vi "Start.vi"(8 "error in (no error)":errorcluster, 9 "Channel Data (DBLs Only)":T1, 10 "Real-Time System Data":T2, 11 "Configuration Data":T3) -> (0 "error out":errorcluster, 1 "Channel Data (DBLs Only)":T1, 2 "Real-Time System Data":T2, 3 "Configuration Data":T3)   [LabVIEW 2014, in "RM interrupt timing Custom Device.lvlib"]
uses:
  RM interrupt timing Custom Device.lvlib
  Configuration Data.ctl
  Real-Time System Data.ctl
  Channel Data.ctl
panel:
  # "Controls"
  # "Indicators"
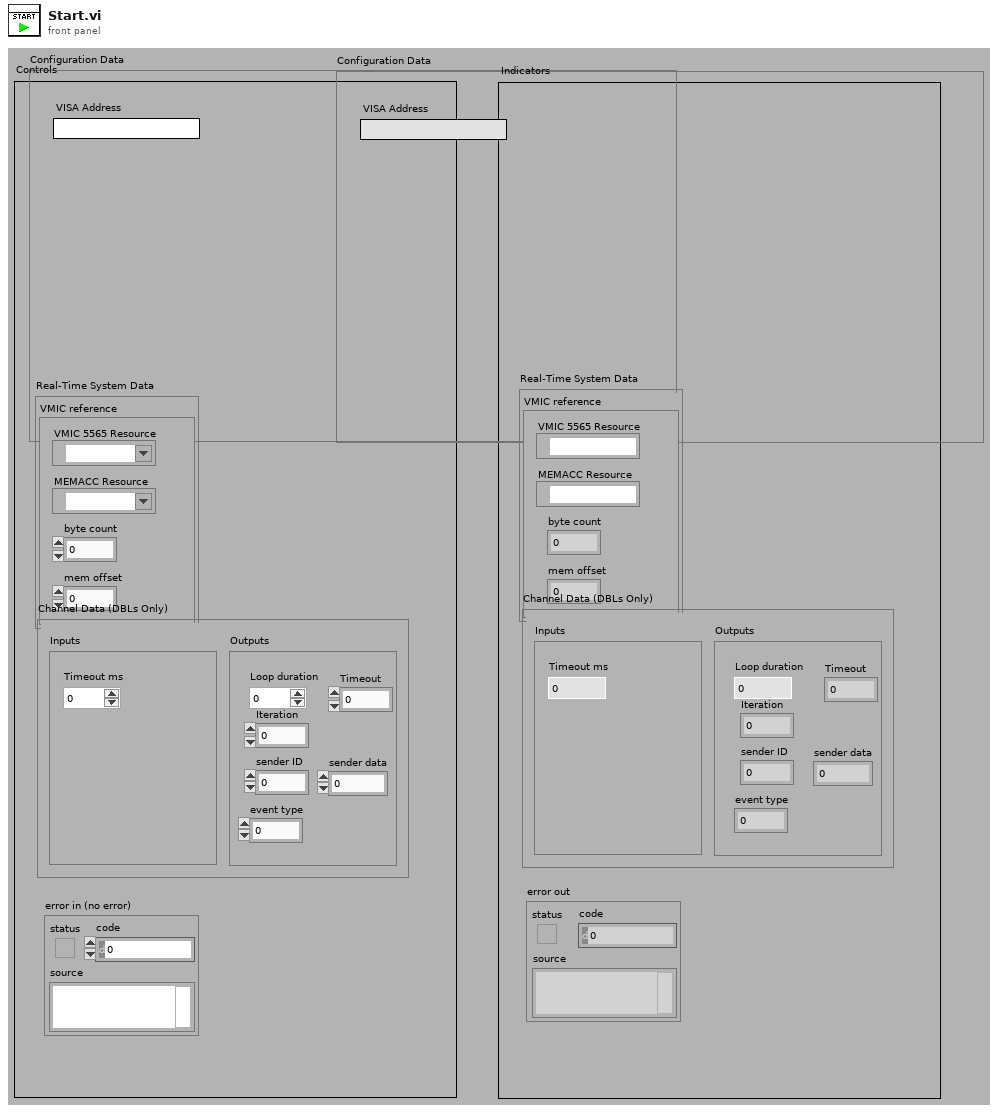
[diagram p1: front panel]
types:
  T1 = typedef "RM interrupt timing Custom Device.lvlib/Channel Data.ctl" = cluster{"Inputs":cluster{"Timeout ms":dbl}, "Outputs":cluster{"Loop duration":dbl, "Iteration":dbl, "Timeout":dbl, "sender data":dbl, "sender ID":dbl, "event type":dbl}}
  T2 = typedef "RM interrupt timing Custom Device.lvlib/Real-Time System Data.ctl" = cluster{"VMIC reference":cluster{"VMIC 5565 Resource":refnum<visa-resource-name>, "MEMACC Resource":refnum<visa-resource-name>, "byte count":u32, "mem offset":u32}}
  T3 = typedef "RM interrupt timing Custom Device.lvlib/Configuration Data.ctl" = cluster{"VISA Address":string}
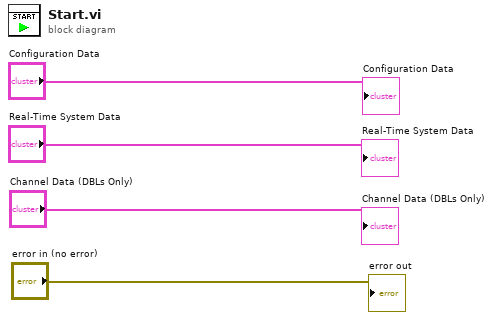
[diagram p0: block diagram]
diagram:
  "error out" <- "error in (no error)"
  "Configuration Data" <- "Configuration Data"
  "Real-Time System Data" <- "Real-Time System Data"
  "Channel Data (DBLs Only)" <- "Channel Data (DBLs Only)"
